vi "Offset_decoder_with_sign.vi"(11 "Array In1":i8[](array[numeric])) -> (2 "CH1":dbl, 3 "CH0":dbl)   [LabVIEW 2012]
panel:
  out "CH1 3":u8 format="%x"
  out "CH1 2":u8 format="%x"
  out "CH1 1":u8 format="%x"
  out "CH1 0":u8 format="%x"
  out "CH0 3":u8 format="%x"
  out "CH0 2":u8 format="%x"
  out "CH0 1":u8 format="%x"
  out "CH0 0":u8 format="%x"
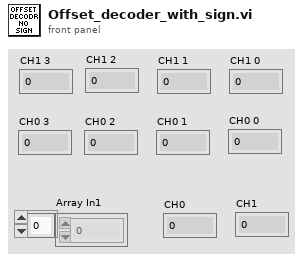
[diagram p1: front panel]
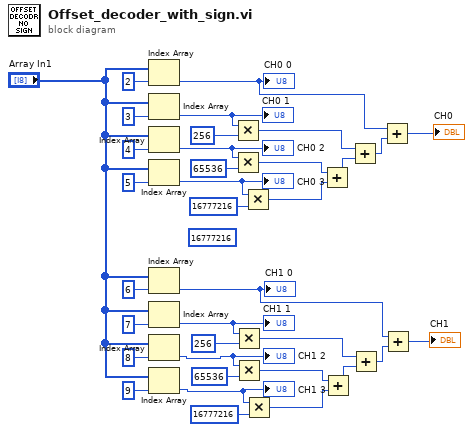
[diagram p0: block diagram]
diagram:
  (unwired) 16777216
  n1 = Index Array(array="Array In1", index=2) -> (element=w20:i8)
  "CH0 0" <- w20
  n2 = Index Array(array="Array In1", index=3) -> (element=w26:i8)
  "CH0 1" <- w26
  n3 = Index Array(array="Array In1", index=4) -> (element=w28:i8)
  "CH0 2" <- w28
  n4 = Index Array(array="Array In1", index=5) -> (element=w30:i8)
  "CH0 3" <- w30
  n5 = Index Array(array="Array In1", index=6) -> (element=w3:i8)
  "CH1 0" <- w3
  n6 = Index Array(array="Array In1", index=7) -> (element=w6:i8)
  "CH1 1" <- w6
  n7 = Index Array(array="Array In1", index=8) -> (element=w4:i8)
  "CH1 2" <- w4
  n8 = Index Array(array="Array In1", index=9) -> (element=w5:i8)
  "CH1 3" <- w5
  n9 = Multiply(x=w26, y=256) -> (x*y=w22:i32)
  n10 = Multiply(x=w28, y=65536) -> (x*y=w25:i32)
  n11 = Multiply(x=w6, y=256) -> (x*y=w8:i32)
  n12 = Multiply(x=w4, y=65536) -> (x*y=w11:i32)
  n13 = Multiply(x=w30, y=16777216) -> (x*y=w24:i32)
  n14 = Multiply(x=w5, y=16777216) -> (x*y=w10:i32)
  n15 = Add(x=w25, y=w24) -> (x+y=w23:i32)
  n16 = Add(x=w11, y=w10) -> (x+y=w9:i32)
  n17 = Add(x=w22, y=w23) -> (x+y=w21:i32)
  n18 = Add(x=w8, y=w9) -> (x+y=w7:i32)
  n19 = Add(x=w20, y=w21) -> (x+y=→"CH0":i32)
  n20 = Add(x=w3, y=w7) -> (x+y=→"CH1":i32)
